vi "Drive_zero_ensemble.vi"(4 "Zero ensemble power in":dbl, 5 "rho0 in":dbl[](array[numeric]), 6 "rho0 decay in":dbl[](array[numeric]), 7 "Zero ensemble in":dbl[](array[numeric]), 8 "Drive Zero Ensemble Up":bool, 9 "Microwave on":bool, 10 "Drive Zero Ensemble Down":bool, 11 "Thermal connection":bool) -> (2 "rho0 out":dbl[](array[numeric]), 3 "Zero ensemble out":dbl[](array[numeric]))   [LabVIEW 2018]
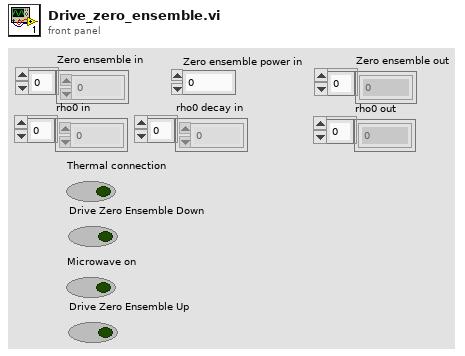
[diagram p1: front panel]
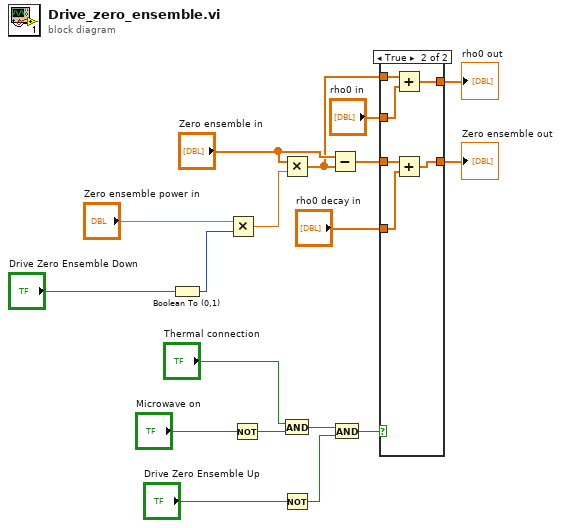
[diagram p0: block diagram]
diagram:
  n1 = Boolean To (0,1)(Boolean="Drive Zero Ensemble Down") -> (0, 1=w1:i16)
  n2 = Multiply(x="Zero ensemble power in", y=w1) -> (x*y=w5:dbl)
  n3 = Not(x="Microwave on") -> (.not. x?=w15:bool)
  n4 = Multiply(x="Zero ensemble in", y=w5) -> (x*y=w3:dbl[])
  n5 = And(x="Thermal connection", y=w15) -> (x .and. y?=w18:bool)
  n6 = Not(x="Drive Zero Ensemble Up") -> (.not. x?=w13:bool)
  n7 = Subtract(x="Zero ensemble in", y=w3) -> (x-y=w2:dbl[])
  n8 = And(x=w18, y=w13) -> (x .and. y?=w12:bool)
  n9 = case shown="True" w12 {
    tunnel: [w19 w21] -> w9
    tunnel: w3 -> [_ w23]
    tunnel: [w20 w22] -> w8
    tunnel: "rho0 in" -> [w20 w24]
    tunnel: "rho0 decay in" -> [_ w25]
    tunnel: w2 -> [w19 w26]
    frame False {
    }
    frame True {
      n10 = Add(x=w23, y=w24) -> (x+y=w22:dbl[])
      n11 = Add(x=w26, y=w25) -> (x+y=w21:dbl[])
    }
  }
  "Zero ensemble out" <- w9
  "rho0 out" <- w8
